vi "Log Error.vi"(8 "error in (no error)":errorcluster, 11 "Da Base in":refnum<class "Da Base.lvclass">) -> (0 "error out":errorcluster, 2 "stop actor?":bool=TRUE, 3 "Da Base out":refnum<class "Da Base.lvclass">)   [LabVIEW 2016, in "Da Base.lvclass"]
uses:
  Da Base.lvclass
  <vilib>/Utility/sysdir.llb/System Directory Type.ctl
  Da Base.lvclass/Da Base.ctl
  <vilib>/Utility/error.llb/DialogType.ctl
  Read Name.vi
  Read Report error and stop.vi
  <vilib>/Utility/error.llb/Error Cluster From Error Code.vi
  <vilib>/ErrorRing/Error Ring.xnode
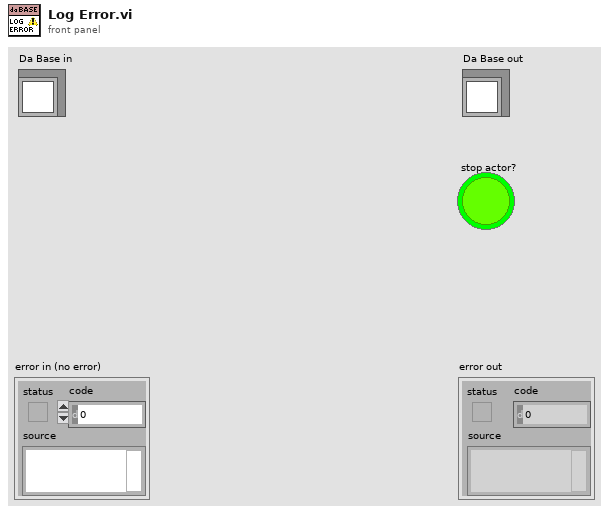
[diagram p1: front panel]
types:
  T1 = enum16{"open", "replace", "create", "open or create", "replace or create", "replace or create with confirmation"}
  T2 = typedef "System Directory Type.ctl" = i32
  T3 = typedef "DialogType.ctl" = u16
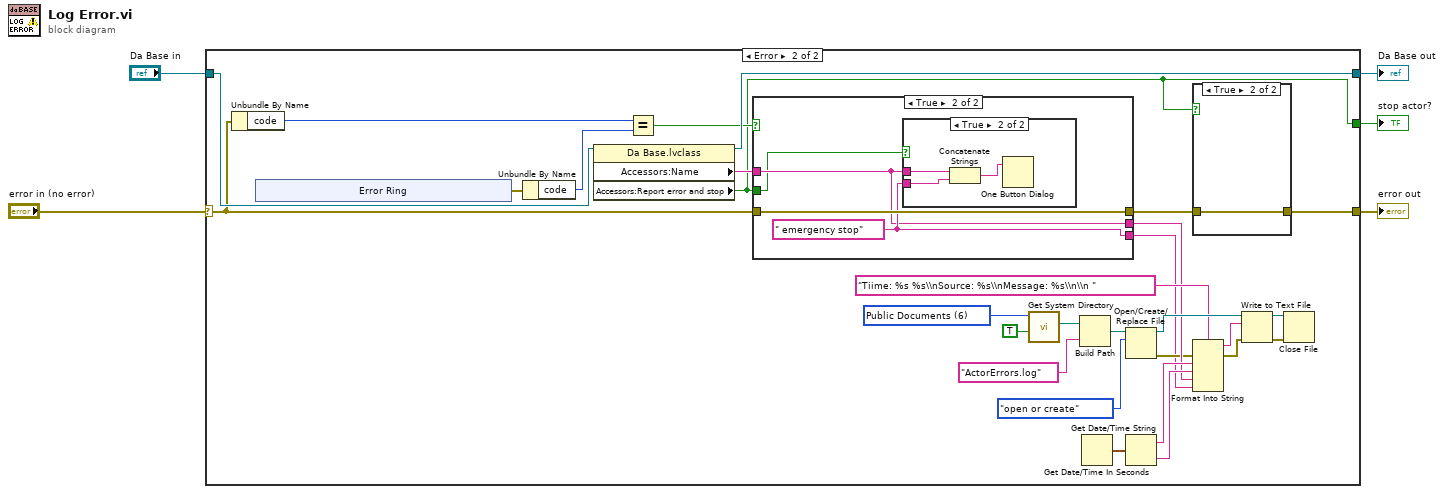
[diagram p0: block diagram]
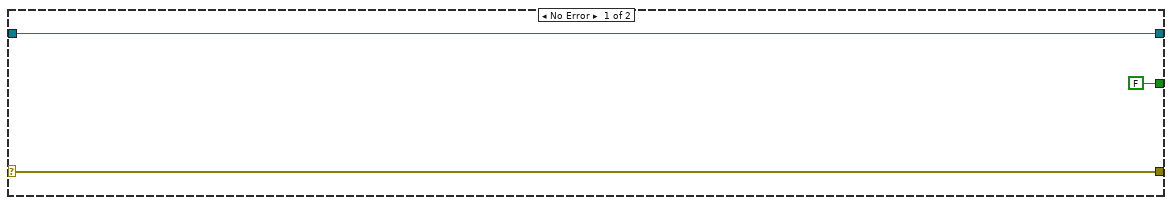
[diagram p2: hidden frame]
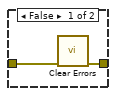
[diagram p3: hidden frame]
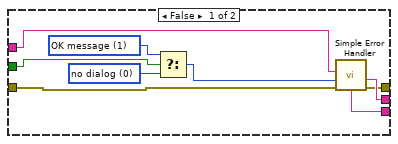
[diagram p4: hidden frame]
diagram:
  n1 = case shown="Error" "error in (no error)" {
    selector: "error in (no error)" -> [w7 w34]
    tunnel: [w7 w10] -> w4
    tunnel: [w8 w36] -> w2
    tunnel: "Da Base in" -> [w8 w37]
    tunnel: [FALSE ("Accessors:Report error and stop") w9] -> w1
    frame No Error {
    }
    frame Error {
      w29 = T2 6 items=["User Home"=0, "User Desktop"=1, "User Documents"=2, "User Application Data"=3, "User Preferences"=4, "User Temporary"=5, "Public Documents"=6, "Public Application Data"=7, "Public Preferences"=8, "Public Cache"=13, "System Core Libraries"=9, "System Installed Libraries"=10, "Application Files"=11, "Boot Volume Root"=12] ("system directory type")
      n2 = Unbundle By Name(w34) -> ("code"=w33:i32)
      n3 = xnode "Error Ring"() -> ("error out"=w35:errorcluster)
      n4 = Unbundle By Name(w35) -> ("code"=w32:i32)
      n5 = property class="Da Base.lvclass"(reference=w37) -> (reference out=w36:refnum<class "Da Base.lvclass">, "Accessors:Name"=w31:string, "Accessors:Report error and stop"=w9:bool)  [unwired: 1 in, 1 out]
      n6 = Equal?(x=w33, y=w32) -> (x = y?=w30:bool)
      n7 = case shown="True" w30 {
        tunnel: w34 -> [w49 w53]
        tunnel: w31 -> [w48 w51]
        tunnel: [w45 w52] -> w12
        tunnel: [w47 w51] -> w18
        tunnel: [w46 w53] -> w11
        tunnel: w9 -> [w44 w50]
        frame False {
          w42 = T3 1 items=["no dialog", "OK message", "continue or stop message", "OK message + warnings", "continue/stop + warnings"] ("type of dialog (OK msg:1)")
          w43 = T3 0 items=["no dialog", "OK message", "continue or stop message", "OK message + warnings", "continue/stop + warnings"] ("type of dialog (OK msg:1)")
          n8 = Select(t=w42, s=w44, f=w43) -> (s? t:f=w41:T3)
          n9 = call <vilib>:"Simple Error Handler.vi"("error source (\" \")"=w48, "type of dialog (OK msg:1)"=w41, "error in (no error)"=w49) -> ("source out"=w47:string, "error out"=w46:errorcluster, "message"=w45:string)  [unwired: 2 in, 2 out]
        }
        frame True {
          w52 = " emergency stop" ("string")
          n10 = case shown="True" w50 {
            tunnel: w52 -> [_ w55]
            tunnel: w51 -> [_ w54]
            frame False {
            }
            frame True {
              n11 = Concatenate Strings(w54, w55) -> (w56:string)
              n12 = One Button Dialog(message=w56) -> ()  [unwired: 1 in, 1 out]
            }
          }
        }
      }
      n13 = call <vilib>:"Get System Directory.vi"("create directory if not found? (F)"=TRUE, "system directory type"=w29) -> ("system directory"=w27:path)  [unwired: 9 in]
      n14 = Build Path(base path=w27, name or relative path="ActorErrors.log") -> (appended path=w25:path)
      n15 = Get Date/Time In Seconds() -> (seconds since 1Jan1904=w21:timestamp)
      n16 = Open/Create/Replace File(file path (use dialog)=w25, operation (0:open)=T1."open or create") -> (refnum out=w23:refnum<file>, error out=w17:errorcluster)  [unwired: 4 in, 1 out]
      n17 = Get Date/Time String(seconds (now)=w21) -> (date string=w20:string, time string=w19:string)  [unwired: 2 in]
      n18 = case shown="True" w9 {
        tunnel: w11 -> [w39 w40]
        tunnel: [w38 w40] -> w10
        frame False {
          n19 = call <vilib>:"Clear Errors.vi"("error in (no error)"=w39) -> ("error out"=w38:errorcluster)  [unwired: 5 in, 1 out]
        }
        frame True {
        }
      }
      n20 = Format Into String(format string="Tiime: %s %s\\nSource: %s\\nMessage: %s\\n\\n ", error in=w17, w20, w19, w18, w12) -> (resulting string=w13:string, error out=w16:errorcluster)  [unwired: 1 in]
      n21 = Write to Text File(file (use dialog)=w23, text=w13, error in=w16) -> (refnum out=w15:refnum<file>, error out=w14:errorcluster)  [unwired: 1 in, 1 out]
      n22 = Close File(refnum=w15, error in=w14) -> ()  [unwired: 2 out]
    }
  }
  "error out" <- w4
  "Da Base out" <- w2
  "stop actor?" <- w1
